vi "Main.vi"(10 "DAQ Type":enum16{"Hardware", "Simulation"}(ring), 11 "Module Admin":refnum<class "Delacor_lib_QMH_Module Admin.lvclass">) -> ()   [LabVIEW 2016, in "Oscilloscope.lvlib"]
doc: "This template is based off of the Queued Message Handler design pattern and the Queued Message Handler project template that ships with LabVIEW.\n\nThe main difference is that the queue is private to this module and communication between modules is performed via Broadcast and Request events.\n\nRequest events are wrapped in public API methods and are handled in the Event Handling Loop (EHL) of this VI. Any module can register for Broadcast events sent by this module. The EHL generates messages based on user interface actions.\n\nThe Message Handling Loop (MHL) processes messages generated by the EHL, or by other messages. The messages are string values, so new messages can be added easily to the Message Cases case structure in the MHL. Each message cluster can also provide an optional value for Message Data, which is a variant that can be converted to whatever message-specific data is required.\n_____\nBased on DQMH Project Template 6.1.0.94."
uses:
  Oscilloscope.lvlib
  <vilib>/Delacor/Delacor QMH/Libraries/Module Admin_class/Delacor_lib_QMH_Module Admin.lvclass
  Class/Agilent 3054A/Agilent 3054A.lvclass
  D:/common_ATE/Libraries/Oscilloscope/Class/Abstract/Abstract.lvclass
  Message Data.ctl
  Class/Abstract/Abstract.lvclass
  Module Data--cluster.ctl
  Scope Config Setting.ctl
  <vilib>/Delacor/Delacor QMH/Libraries/Message Queue_class/Delacor_lib_QMH_Message Queue.lvclass/Delacor_lib_QMH_Message Queue.ctl
  Stop Argument--cluster.ctl
  <vilib>/Delacor/Delacor QMH/Libraries/Module Admin_class/Delacor_lib_QMH_Module Admin.lvclass/Delacor_lib_QMH_Module Admin.ctl
  REQ Initialize Hardware Argument--cluster.ctl
  REQ Initialize Hardware (Reply Payload)--cluster.ctl
  REQ Auto setup Argument--cluster.ctl
  Close Ref Argument--cluster.ctl
  Acquire Waveform Argument--cluster.ctl
  Acquire Waveform (Reply Payload)--cluster.ctl
  REQ Channel Setting Argument--cluster.ctl
  REQ Configure DVM Argument--cluster.ctl
  REQ Read DVM Argument--cluster.ctl
  REQ Read DVM (Reply Payload)--cluster.ctl
  REQ Acq Waveform Argument--cluster.ctl
  REQ Retry Oscilloscope Argument--cluster.ctl
  <vilib>/Utility/miscctls.llb/LVPointTypeDef.ctl
  User Interface/Instrument Address Command.ctl
  <vilib>/Delacor/Delacor QMH/Libraries/Message Queue_class/Delacor_lib_QMH_Enqueue Message (Single).vi
  <vilib>/Delacor/Delacor QMH/Libraries/Module Admin_class/Delacor_lib_QMH_Get External Launch.vi
  <vilib>/Utility/error.llb/Error Cluster From Error Code.vi
  <vilib>/ErrorRing/Error Ring.xnode
  <vilib>/Delacor/Delacor QMH/Libraries/Message Queue_class/Delacor_lib_QMH_Message Queue.lvclass
  User Interface/User Interface.lvlib
  Error Log/Error Log.lvlib
panel:
  out "Channel":i32
  out "Waveform Data":waveform(dbl)(graph)
  out "error out":errorcluster
  out "Status":string
  in  "Simulate MHL Error":bool
  in  "Simulate EHL Error":bool
  # "Other QMH Modules communicate with this Module via its Public API (wrappers for its Request Events).\n\nThis Module communicates with other Modules via its Broadcast Events.\nAny module that wants to get these messages, just registers for this module's Broadcast events."
  # "This template is for the Delacor Modified Queued Message Handler design pattern.\n\nSee the block diagram for more information on how to use this template."
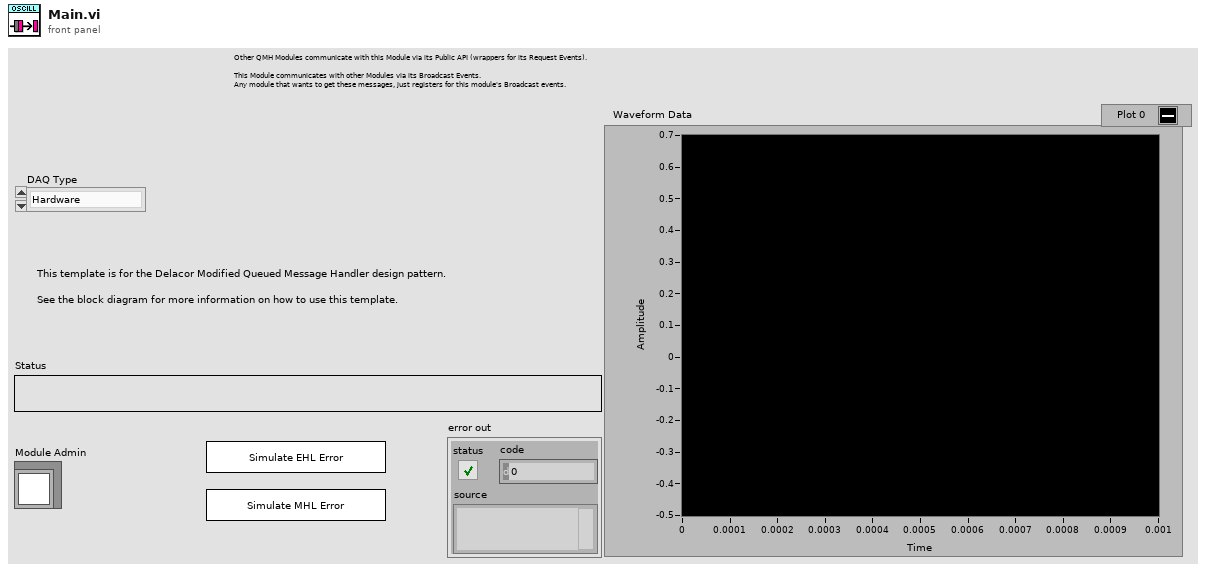
[diagram p1: front panel]
types:
  T1 = typedef "Oscilloscope.lvlib/Message Data.ctl" = cluster{"Message":string, "Data":waveform(dbl)}
  T2 = typedef "Oscilloscope.lvlib/Request Events--cluster.ctl" = cluster{"Stop Module":refnum<user-event>, "Show Panel":refnum<user-event>, "Hide Panel":refnum<user-event>, "Get Module Execution Status":refnum<user-event>, "Show Diagram":refnum<user-event>, "REQ Initialize Hardware":refnum<user-event>, "REQ Auto setup":refnum<user-event>, "Close Ref":refnum<user-event>, "Acquire Waveform":refnum<user-event>, "REQ Channel Setting":refnum<user-event>, "REQ Configure DVM":refnum<user-event>, "REQ Read DVM":refnum<user-event>, "REQ Acq Data":refnum<user-event>, "REQ Wakeup_helper_loop":refnum<user-event>, "REQ Acq Waveform":refnum<user-event>, "REQ Retry Oscilloscope":refnum<user-event>}
  T3 = enum32{"invalid lock state", "Not Locked", "Locked (No Password)", "Password-protected"}
  T4 = typedef "Oscilloscope.lvlib/Stop Argument--cluster.ctl" = cluster{"Origin":string, "Exit via Stop Module Req?":bool, "Wait for Module to stop?":bool}
  T5 = typedef "Oscilloscope.lvlib/REQ Initialize Hardware Argument--cluster.ctl" = cluster{"Connection Ref":variant, "Wait Notifier":refnum<notifier>, "wait for reply":bool}
  T6 = typedef "Oscilloscope.lvlib/REQ Auto setup Argument--cluster.ctl" = cluster{"Boolean":bool}
  T7 = typedef "Oscilloscope.lvlib/Close Ref Argument--cluster.ctl" = cluster{"Boolean":bool}
  T8 = typedef "Oscilloscope.lvlib/Acquire Waveform Argument--cluster.ctl" = cluster{"Channel":i32, "Wait Notifier":refnum<notifier>, "wait for reply":bool}
  T9 = typedef "Oscilloscope.lvlib/REQ Channel Setting Argument--cluster.ctl" = cluster{"Channel Setting":cluster{"Channel Name (0: Channel 1)":i32, "Coupling (1: DC)":i32, "Vertical Offset (0.0)":dbl, "Vertical Range (40.0 V)":dbl, "Probe Attenuation (1.0)":dbl, "Enable Channel (T: Enable)":bool, "Impedance (0: 1 MOhm)":i32, "Vertical Scale (5.0 V)":dbl, "Vertical Setting (1: Vertical Range)":i32}}
  T10 = typedef "Oscilloscope.lvlib/REQ Configure DVM Argument--cluster.ctl" = cluster{"DVM Setting":cluster{"DVM Channel":i32, "Enable DVM Analysis":bool, "Auto Range ":bool, "DVM Type":i32}}
  T11 = typedef "Oscilloscope.lvlib/REQ Read DVM Argument--cluster.ctl" = cluster{"Wait Notifier":refnum<notifier>, "wait for reply":bool}
  T12 = typedef "Oscilloscope.lvlib/REQ Acq Waveform Argument--cluster.ctl" = cluster{"Boolean":bool, "Channel":i32}
  T13 = typedef "Oscilloscope.lvlib/REQ Retry Oscilloscope Argument--cluster.ctl" = cluster{"Boolean":bool}
  T14 = typedef "User Interface.lvlib/Instrument Address Command.ctl" = enum16{"Init", "Read", "Write", "Close"}
  T15 = typedef "LVPointTypeDef.ctl" = cluster{"Horizontal":i16, "Vertical":i16}
  T16 = enum32{"Invalid", "Standard", "Closed", "Hidden", "Minimized", "Maximized"}
  T17 = typedef "Oscilloscope.lvlib/REQ Initialize Hardware (Reply Payload)--cluster.ctl" = cluster{"Connect?":bool, "error":errorcluster}
  T18 = typedef "Oscilloscope.lvlib/REQ Read DVM (Reply Payload)--cluster.ctl" = cluster{"3-digit DVM":dbl, "5-digit Frequency":dbl, "error":errorcluster}
  T19 = typedef "Oscilloscope.lvlib/Module Data--cluster.ctl" = cluster{"Status":string, "Abstract.lvclass":refnum<class "Abstract.lvclass">, "Inst_Path":path, "Scope":T20}
  T20 = typedef "Oscilloscope.lvlib/Scope Config Setting.ctl" = cluster{"Connection":cluster{"Ref":variant}, "Channel Setting":cluster{"Channel Name (0: Channel 1)":i32, "Coupling (1: DC)":i32, "Vertical Offset (0.0)":dbl, "Vertical Range (40.0 V)":dbl, "Probe Attenuation (1.0)":dbl, "Enable Channel (T: Enable)":bool, "Impedance (0: 1 MOhm)":i32, "Vertical Scale (5.0 V)":dbl, "Vertical Setting (1: Vertical Range)":i32}}
  T21 = cluster{"Channel Name (0: Channel 1)":i32, "Coupling (1: DC)":i32, "Vertical Offset (0.0)":dbl, "Vertical Range (40.0 V)":dbl, "Probe Attenuation (1.0)":dbl, "Enable Channel (T: Enable)":bool, "Impedance (0: 1 MOhm)":i32, "Vertical Scale (5.0 V)":dbl, "Vertical Setting (1: Vertical Range)":i32}
  T22 = cluster{"DVM Channel":i32, "Enable DVM Analysis":bool, "Auto Range ":bool, "DVM Type":i32}
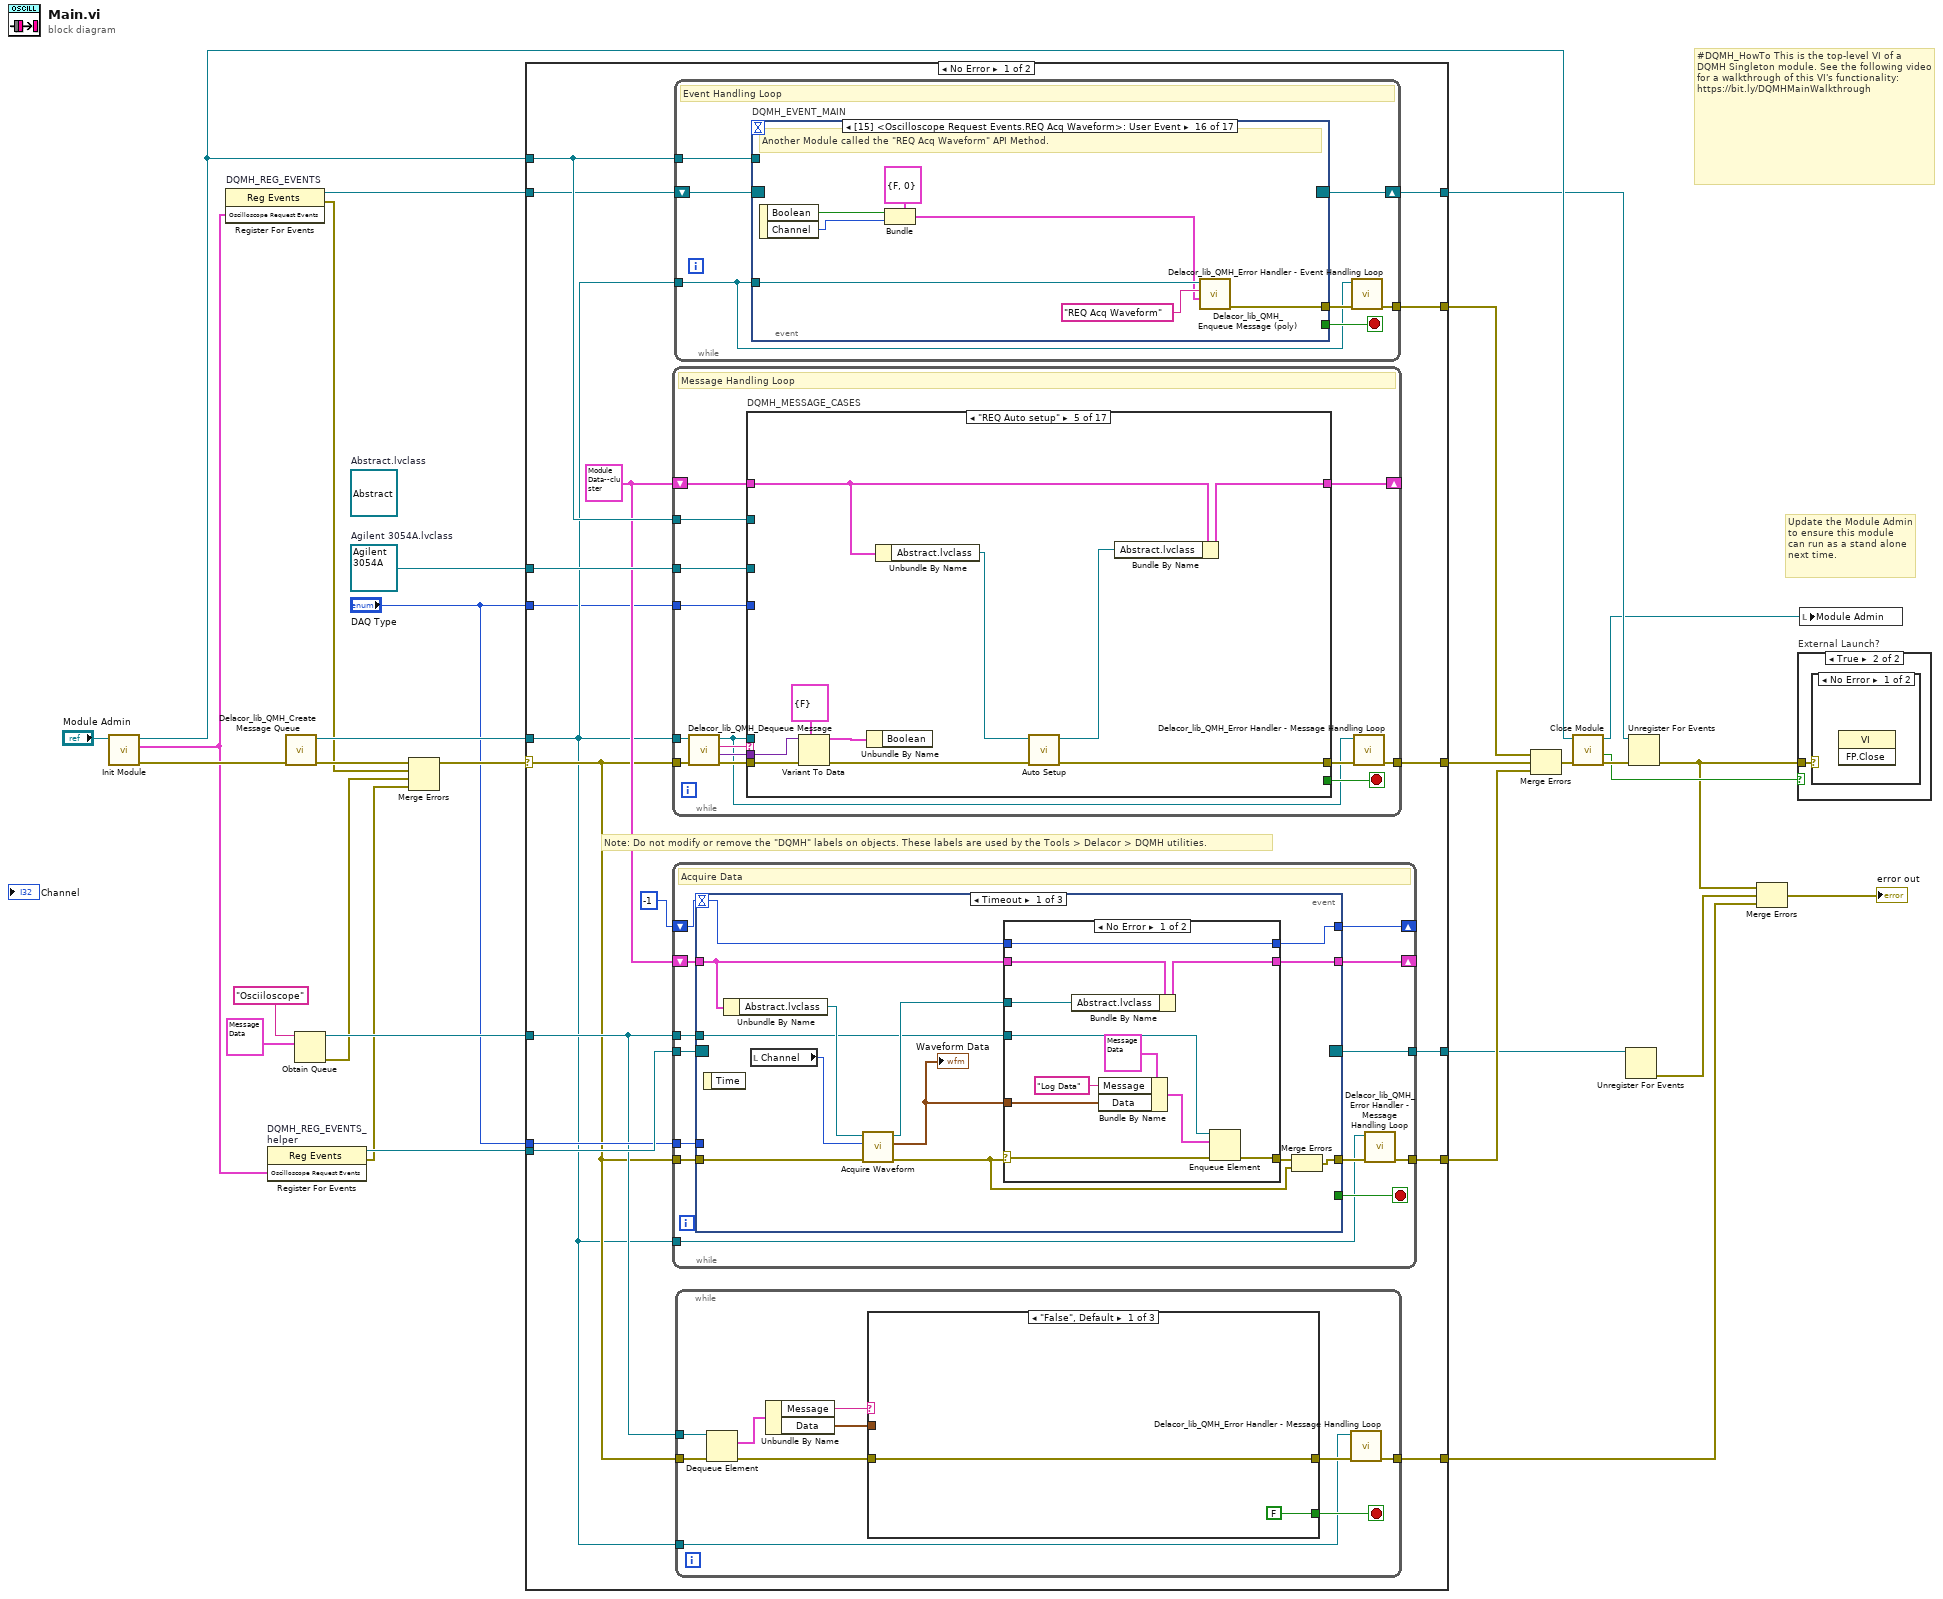
[diagram p0: block diagram]
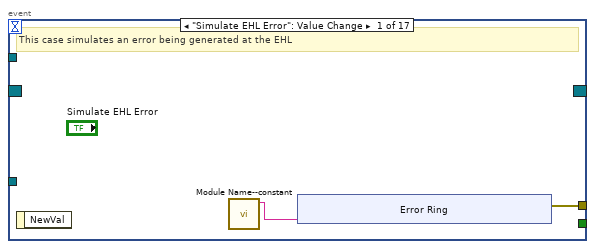
[diagram p2: hidden frame]
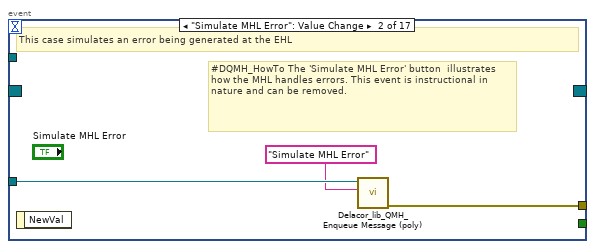
[diagram p3: hidden frame]
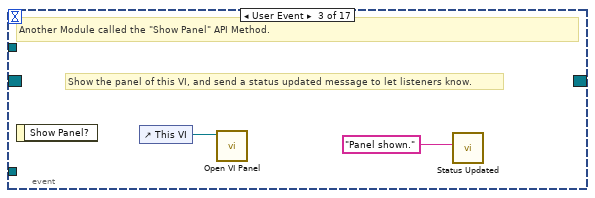
[diagram p4: hidden frame]
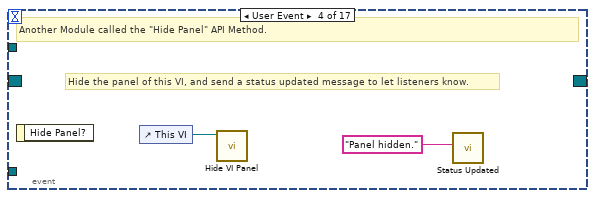
[diagram p5: hidden frame]
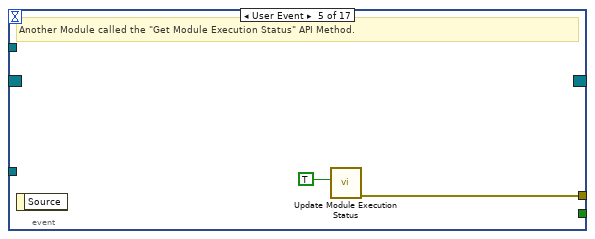
[diagram p6: hidden frame]
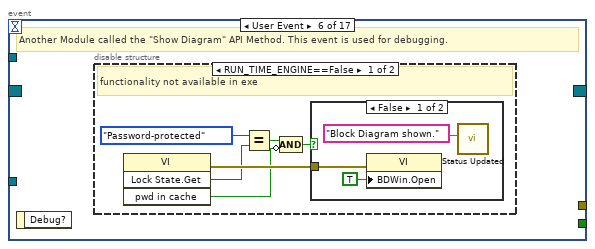
[diagram p7: hidden frame]
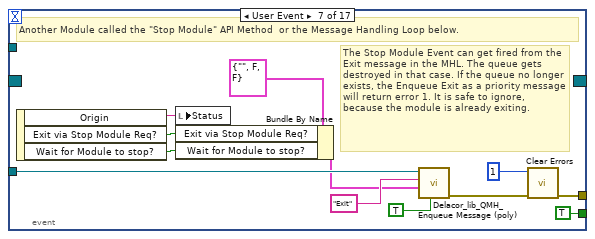
[diagram p10: hidden frame]
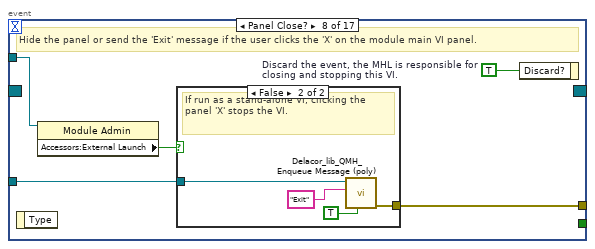
[diagram p11: hidden frame]
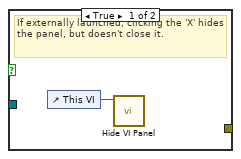
[diagram p12: hidden frame]
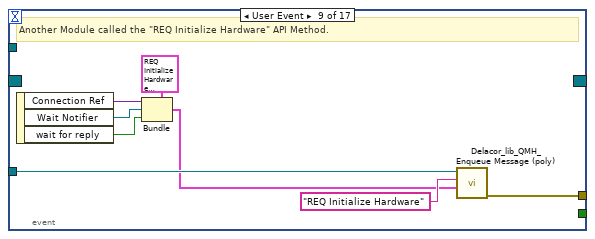
[diagram p13: hidden frame]
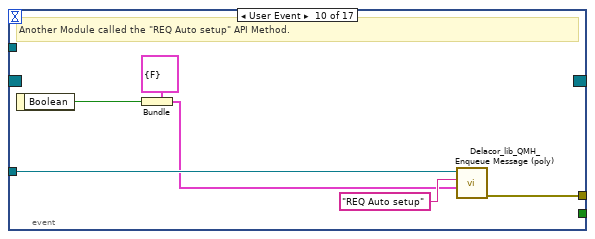
[diagram p14: hidden frame]
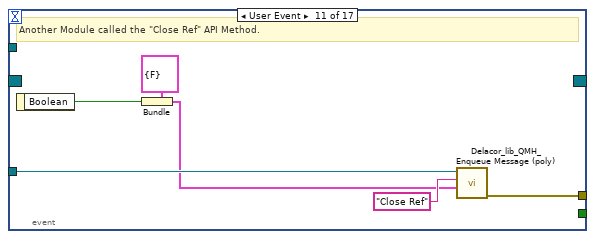
[diagram p15: hidden frame]
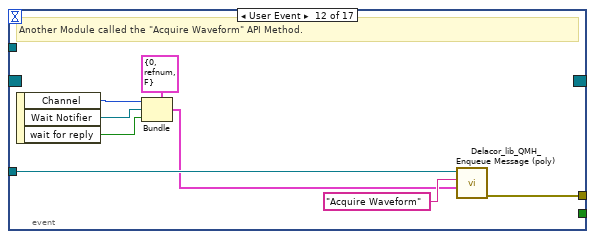
[diagram p16: hidden frame]
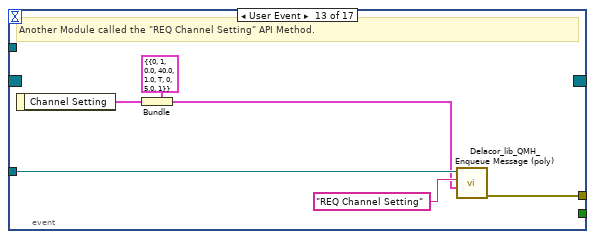
[diagram p17: hidden frame]
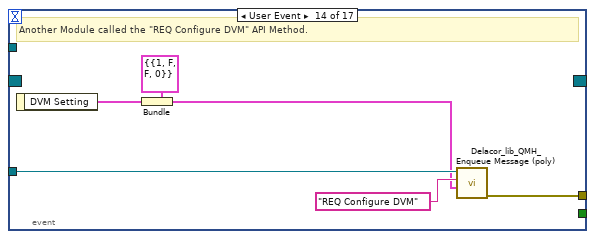
[diagram p18: hidden frame]
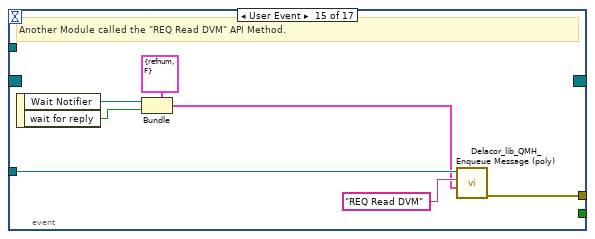
[diagram p19: hidden frame]
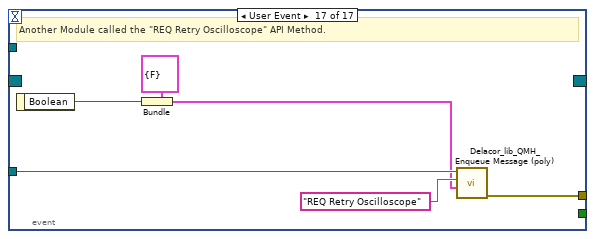
[diagram p20: hidden frame]
diagram:
  w16 = refnum<class "Agilent 3054A.lvclass"> refnum  # Agilent 3054A.lvclass
  (unwired) refnum<class "Abstract.lvclass"> refnum  # Abstract.lvclass
  # "#DQMH_HowTo This is the top-level VI of a DQMH Singleton module. See the following video for a walkthrough of this VI's functionality: https://bit.ly/DQMHMainWalkthrough"
  # "Update the Module Admin to ensure this module can run as a stand alone next time."
  n1 = call "Init Module.vi"("Singleton Module Admin in"="Module Admin") -> ("error out"=w29:errorcluster, "Oscilloscope Request Events"=w15:T2, "Singleton Module Admin out"=w23:refnum<class "Delacor_lib_QMH_Module Admin.lvclass">)  [unwired: 8 in]
  n2 = register-events "DQMH_REG_EVENTS"(w15) -> (reference out=w21:refnum<event-registration>, error out=w8:errorcluster)  [unwired: 2 in]
  n3 = register-events "DQMH_REG_EVENTS_helper"(w15) -> (reference out=w14:refnum<event-registration>, error out=w2:errorcluster)  [unwired: 2 in]
  n4 = call <vilib>:"Delacor_lib_QMH_Create Message Queue.vi"("error in"=w29) -> ("error out"=w25:errorcluster, "Message Queue"=w20:refnum<class "Delacor_lib_QMH_Message Queue.lvclass">)  [unwired: 9 in]
  n5 = Obtain Queue(name (unnamed)="Osciiloscope", element data type=T1 {"Message"="", "Data"={"t0"=timestamp(0 s since 1904-01-01), "dt"=1.0, "Y"=[]}}) -> (queue out=w5:refnum<queue>, error out=w3:errorcluster)  [unwired: 3 in, 1 out]
  n6 = Merge Errors(w25, w8, w3, w2) -> (w24:errorcluster)
  n7 = case shown="No Error" w24 {
    selector: w24 -> [w33 w461]
    tunnel: [w47 w460] -> w30
    tunnel: [w46 _] -> w27
    tunnel: w23 -> [w45 w464]
    tunnel: [w44 w463] -> w22
    tunnel: w21 -> [w43 w463]
    tunnel: w20 -> [w32 w462]
    tunnel: w16 -> [w42 _]
    tunnel: w14 -> [w40 _]
    tunnel: [w39 _] -> w13
    tunnel: [w38 _] -> w11
    tunnel: "DAQ Type" -> [w36 _]
    tunnel: w5 -> [w35 _]
    tunnel: [w34 _] -> w4
    tunnel: "DAQ Type" -> [w31 _]
    frame No Error {
      w37 = T19 {"Status"="", "Abstract.lvclass"=refnum, "Inst_Path"=path "", "Scope"={"Connection"={"Ref"=variant}, "Channel Setting"={"Channel Name (0: Channel 1)"=0, "Coupling (1: DC)"=1, "Vertical Offset (0.0)"=0.0, "Vertical Range (40.0 V)"=40.0, "Probe Attenuation (1.0)"=1.0, "Enable Channel (T: Enable)"=TRUE, "Impedance (0: 1 MOhm)"=0, "Vertical Scale (5.0 V)"=5.0, "Vertical Setting (1: Vertical Range)"=1}}} ("Data Cluster")
      # "Note: Do not modify or remove the \"DQMH\" labels on objects. These labels are used by the Tools > Delacor > DQMH utilities."
      n8 = while {
        tunnel: w32 -> [w168]
        shift-right: [w172] -> _
        shift-left: w37 -> [w173]
        tunnel: w33 -> [w176]
        tunnel: [w174] -> w47
        tunnel: w45 -> [w166]
        tunnel: w42 -> [w165]
        tunnel: w31 -> [w164]
        stop <- w171 stop-if-true
        # "Message Handling Loop"
        n9 = call-dynamic "Delacor_lib_QMH_Dequeue Message.vi"("error in"=w176, "Message Queue in"=w168) -> ("error out"=w175:errorcluster, "Message Data"=w169:variant, "Message"=w170:string, "Message Queue out"=w167:refnum<class "Delacor_lib_QMH_Message Queue.lvclass">)  [unwired: 6 in]
        n10 = case "DQMH_MESSAGE_CASES" shown="\"REQ Auto setup\"" w170 {
          selector: w170 -> [_ _ _ _ _ _ _ _ _ _ _ _ _ _ _ _ w379]
          tunnel: w167 -> [w184 _ _ _ _ _ _ _ _ _ _ _ _ _ w350 w371 _]
          tunnel: w175 -> [w180 w215 w217 w235 w247 w257 w268 w284 w296 w307 w322 w332 w334 w339 w357 w377 w381]
          tunnel: [w185 w208 w217 w222 w242 w253 w263 w275 w291 w301 w311 w331 w334 w338 w353 w374 w382] -> w177
          tunnel: w173 -> [w194 w214 w216 w227 w241 w252 w261 w274 w290 w300 w318 w330 w333 w336 w352 w370 w380]
          tunnel: [w193 w206 w216 w224 w239 w250 w259 w272 w288 w300 w309 w330 w333 w336 w352 w370 w380] -> w172
          tunnel: [_ _ _ _ _ _ _ _ _ _ _ _ _ _ _ w369 _] -> w171
          tunnel: w169 -> [_ _ _ w234 w245 w256 w267 w283 w295 w306 w321 _ _ _ w351 w368 _]
          tunnel: w166 -> [w195 _ _ _ _ _ _ _ _ _ _ _ _ _ w349 w363 _]
          tunnel: w165 -> [w187 _ _ _ _ _ _ _ _ _ _ _ _ _ _ _ _]
          tunnel: w164 -> [_ _ _ w223 _ _ _ _ _ _ w315 _ _ _ _ _ _]
          frame "Initialize" {
            w189 = "Initial Message" ("Initial Message")
            # "Initialize - Any operation that needs to be done before the module can receive messages. Synchronize Caller Events.vi will inform Start Module.vi that the module has launched and is ready to receive messages. Module Did Init.vi will broadcast that the module initialized."
            n11 = call "Synchronize Caller Events.vi"("error in (no error)"=w180, "Singleton Module Admin in"=w195) -> ("error out"=w183:errorcluster, "Singleton Module Admin out"=w190:refnum<class "Delacor_lib_QMH_Module Admin.lvclass">)  [unwired: 8 in]
            n12 = property class="Module Admin"(reference=w190) -> ("Accessors:External Launch"=w199:bool)  [unwired: 1 in, 2 out]
            n13 = property on="Pane" class="Pane"("Origin"=T15 {"Horizontal"=0, "Vertical"=0}) -> ()  [unwired: 2 in, 2 out]
            n14 = call "Module Name--constant.vi"() -> ("Module Name"=w191:string)  [unwired: 11 in]
            n15 = call "Module Did Init.vi"("error in (no error)"=w183, "Initialized?"=TRUE, "Origin"=w191) -> ()  [unwired: 8 in, 1 out]
            n16 = call "Instrument Address.vi"("Command"=Instrument_Address_Command."Init", "error in (no error)"=w180, "name or relative path"="Instrument.ini") -> ("error out"=w179:errorcluster, "path_out"=w178:path)  [unwired: 6 in, 1 out]
            n17 = Select(t=T16."Hidden" ("State"), s=w199, f=T16."Standard" ("State")) -> (s? t:f=w196:T16)
            n18 = call "Module Name--constant.vi"() -> ("Module Name"=w202:string)  [unwired: 11 in]
            n19 = property class="VI"("Front Panel.Title"=w202) -> (reference out=w201:refnum<vi>, error out=w204:errorcluster)  [unwired: 2 in]
            n20 = Bundle By Name(cluster=w194, "Status"=w189, "Abstract.lvclass"=w187, "Inst_Path"=w178) -> (w193:T19)
            n21 = invoke class="VI" method="FP.Open"(reference=w201, error in=w204, "State"=w196) -> (reference out=w200:refnum<vi>, error out=w203:errorcluster)  [unwired: 2 in, 3 out]
            n22 = call-poly <vilib>:"Delacor_lib_QMH_Enqueue Message (poly).vi"("error in"=w179, "Message"="REQ Inst Address", "Message Queue in"=w184) -> ("error out"=w185:errorcluster)  [unwired: 7 in, 1 out]
            n23 = invoke class="VI" method="FP.Center"(reference=w200, error in=w203) -> ()  [unwired: 1 in, 3 out]
            "Status" <- w189
          }
          frame "REQ Inst Address" {
            n24 = Unbundle By Name(w214) -> ("Inst_Path"=w212:path)
            n25 = call "Instrument Address.vi"("Command"=Instrument_Address_Command."Read", "error in (no error)"=w215, "path_in"=w212) -> ("error out"=w209:errorcluster, "Instrument Parameter"=w211:string[][])  [unwired: 6 in, 1 out]
            n26 = Index Array(array=w211, index (row)=3) -> (element=w207:string[])  [unwired: 1 in]
            n27 = call "Update Inst Config.vi"("error in (no error)"=w209, "Data In"=w207) -> ("error out"=w208:errorcluster, "Scope"=w205:T20)  [unwired: 8 in]
            n28 = Bundle By Name(cluster=w214, "Scope"=w205) -> (w206:T19)
          }
          frame "---Module Specific---" {
            # "Separator -- The following cases handle messages specific to this Module."
          }
          frame "REQ Initialize Hardware" {
            n29 = Variant To Data(error in=w235, type=T5 {"Connection Ref"=variant, "Wait Notifier"=refnum, "wait for reply"=FALSE} ("REQ Initialize Hardware Argument"), Variant=w234) -> (data=w232:T5, error out=w225:errorcluster)
            n30 = Unbundle By Name(w227) -> ("Abstract.lvclass"=w226:refnum<class "Abstract.lvclass">, "Scope.Connection.Ref"=w218:variant)
            n31 = Unbundle By Name(w232) -> ("Wait Notifier"=w231:refnum<notifier>, "wait for reply"=w230:bool)
            n32 = call-dynamic "Initialize Hardware.vi"("error in (no error)"=w225, "DAQ Type"=w223, "Connection Ref"=w218, "Abstract in"=w226) -> ("error out"=w222:errorcluster, "Abstract out"=w219:refnum<class "Abstract.lvclass">)  [unwired: 6 in]
            n33 = Unbundle By Name(w222) -> ("status"=w221:bool)
            n34 = Bundle By Name(cluster=w227, "Abstract.lvclass"=w219) -> (w224:T19)
            n35 = Not(x=w221) -> (.not. x?=w220:bool)
            n36 = Bundle By Name(cluster=T17 {"Connect?"=FALSE, "error"={"status"=FALSE, "code"=0, "source"=""}} ("REQ Initialize Hardware (Reply Payload)"), "Connect?"=w220) -> (w229:T17)
            n37 = case shown="True" w230 {
              tunnel: w231 -> [_ w237]
              tunnel: w229 -> [_ w236]
              frame False {
              }
              frame True {
                n38 = Send Notification(notification=w236, notifier=w237) -> ()  [unwired: 1 in, 2 out]
              }
            }
          }
          frame "REQ Auto setup" {
            n39 = Variant To Data(error in=w247, type=T6 {"Boolean"=FALSE} ("REQ Auto setup Argument"), Variant=w245) -> (data=w243:T6, error out=w246:errorcluster)
            n40 = Unbundle By Name(w243) -> ()  [unwired: 1 out]
            n41 = Unbundle By Name(w241) -> ("Abstract.lvclass"=w240:refnum<class "Abstract.lvclass">)
            n42 = call-dynamic "Auto Setup.vi"("error in (no error)"=w246, "Abstract in"=w240) -> ("error out"=w242:errorcluster, "Abstract out"=w238:refnum<class "Abstract.lvclass">)  [unwired: 8 in]
            n43 = Bundle By Name(cluster=w241, "Abstract.lvclass"=w238) -> (w239:T19)
          }
          frame "REQ Channel Setting" {
            n44 = Variant To Data(error in=w257, type=T9 {"Channel Setting"={"Channel Name (0: Channel 1)"=0, "Coupling (1: DC)"=1, "Vertical Offset (0.0)"=0.0, "Vertical Range (40.0 V)"=40.0, "Probe Attenuation (1.0)"=1.0, "Enable Channel (T: Enable)"=TRUE, "Impedance (0: 1 MOhm)"=0, "Vertical Scale (5.0 V)"=5.0, "Vertical Setting (1: Vertical Range)"=1}} ("REQ Channel Setting Argument"), Variant=w256) -> (error out=w254:errorcluster)  [unwired: 1 out]
            n45 = Unbundle By Name(w252) -> ("Abstract.lvclass"=w251:refnum<class "Abstract.lvclass">, "Scope.Channel Setting"=w248:T21)
            n46 = call-dynamic "Configure Channel.vi"("error in (no error)"=w254, "Channel Setting"=w248, "Abstract in"=w251) -> ("error out"=w253:errorcluster, "Abstract out"=w249:refnum<class "Abstract.lvclass">)  [unwired: 7 in]
            n47 = Bundle By Name(cluster=w252, "Abstract.lvclass"=w249) -> (w250:T19)
          }
          frame "REQ Configure DVM" {
            n48 = Variant To Data(error in=w268, type=T10 {"DVM Setting"={"DVM Channel"=1, "Enable DVM Analysis"=FALSE, "Auto Range "=FALSE, "DVM Type"=0}} ("REQ Configure DVM Argument"), Variant=w267) -> (data=w265:T10, error out=w264:errorcluster)
            n49 = Unbundle By Name(w265) -> ("DVM Setting"=w262:T22)
            n50 = Unbundle By Name(w261) -> ("Abstract.lvclass"=w260:refnum<class "Abstract.lvclass">)
            n51 = call-dynamic "Configure DVM Setting.vi"("error in (no error)"=w264, "DVM Setting"=w262, "Abstract in"=w260) -> ("error out"=w263:errorcluster, "Abstract out"=w258:refnum<class "Abstract.lvclass">)  [unwired: 7 in]
            n52 = Bundle By Name(cluster=w261, "Abstract.lvclass"=w258) -> (w259:T19)
          }
          frame "REQ Read DVM" {
            n53 = Variant To Data(error in=w284, type=T11 {"Wait Notifier"=refnum, "wait for reply"=FALSE} ("REQ Read DVM Argument"), Variant=w283) -> (data=w281:T11, error out=w276:errorcluster)
            n54 = Unbundle By Name(w281) -> ("Wait Notifier"=w280:refnum<notifier>, "wait for reply"=w279:bool)
            n55 = Unbundle By Name(w274) -> ("Abstract.lvclass"=w273:refnum<class "Abstract.lvclass">)
            n56 = call-dynamic "Read DVM.vi"("error in (no error)"=w276, "Abstract in"=w273) -> ("error out"=w275:errorcluster, "5-digit Frequency"=w269:dbl, "3-digit DVM"=w270:dbl, "Abstract out"=w271:refnum<class "Abstract.lvclass">)  [unwired: 6 in]
            n57 = Bundle By Name(cluster=T18 {"3-digit DVM"=0.0, "5-digit Frequency"=0.0, "error"={"status"=FALSE, "code"=0, "source"=""}} ("REQ Read DVM (Reply Payload)"), "3-digit DVM"=w270, "5-digit Frequency"=w269) -> (w278:T18)
            n58 = Bundle By Name(cluster=w274, "Abstract.lvclass"=w271) -> (w272:T19)
            n59 = case shown="True" w279 {
              tunnel: w280 -> [_ w286]
              tunnel: w278 -> [_ w285]
              frame False {
              }
              frame True {
                n60 = Send Notification(notification=w285, notifier=w286) -> ()  [unwired: 1 in, 2 out]
              }
            }
          }
          frame "Close Ref" {
            n61 = Variant To Data(error in=w296, type=T7 {"Boolean"=FALSE} ("Close Ref Argument"), Variant=w295) -> (data=w293:T7, error out=w292:errorcluster)
            n62 = Unbundle By Name(w290) -> ("Abstract.lvclass"=w289:refnum<class "Abstract.lvclass">)
            n63 = Unbundle By Name(w293) -> ()  [unwired: 1 out]
            n64 = call-dynamic "Close Ref.vi"("error in (no error)"=w292, "Abstract in"=w289) -> ("error out"=w291:errorcluster, "Abstract out"=w287:refnum<class "Abstract.lvclass">)  [unwired: 8 in]
            n65 = Bundle By Name(cluster=w290, "Abstract.lvclass"=w287) -> (w288:T19)
          }
          frame "REQ Acq Waveform" {
            n66 = Variant To Data(error in=w307, type=T12 {"Boolean"=FALSE, "Channel"=0} ("REQ Acq Waveform Argument"), Variant=w306) -> (data=w304:T12, error out=w303:errorcluster)
            n67 = Unbundle By Name(w300) -> ("Abstract.lvclass"=w299:refnum<class "Abstract.lvclass">)
            n68 = Unbundle By Name(w304) -> ("Channel"=w302:i32)
            n69 = To Variant(anything=w299) -> (Variant=w297:variant)
            n70 = call "REQ Wakeup_helper_loop.vi"("error in"=w303, "Channel"=w302, "Timeout"=0, "Data"=w297) -> ("error out"=w301:errorcluster)  [unwired: 7 in]
          }
          frame "REQ Retry Oscilloscope" {
            n71 = Unbundle By Name(w318) -> ("Abstract.lvclass"=w317:refnum<class "Abstract.lvclass">, "Scope.Connection.Ref"=w316:variant)
            n72 = Variant To Data(error in=w322, type=T13 {"Boolean"=FALSE} ("REQ Retry Oscilloscope Argument"), Variant=w321) -> (error out=w319:errorcluster)  [unwired: 1 out]
            n73 = call-dynamic "Initialize Hardware.vi"("error in (no error)"=w319, "DAQ Type"=w315, "Connection Ref"=w316, "Abstract in"=w317) -> ("error out"=w310:errorcluster, "Abstract out"=w308:refnum<class "Abstract.lvclass">)  [unwired: 6 in]
            n74 = local read "Channel"() -> (w313:i32)
            n75 = Bundle By Name(cluster=w318, "Abstract.lvclass"=w308) -> (w309:T19)
            n76 = case shown="No Error" w310 {
              selector: w310 -> [w327 _]
              tunnel: [w328 w329] -> w314
              tunnel: w308 -> [w326 _]
              tunnel: w313 -> [w325 _]
              frame No Error {
                n77 = To Variant(anything=w326) -> (Variant=w323:variant)
                n78 = call "REQ Wakeup_helper_loop.vi"("error in"=w327, "Channel"=w325, "Timeout"=0, "Data"=w323) -> ("error out"=w328:errorcluster)  [unwired: 7 in]
              }
              frame Error {
                n79 = call "REQ Retry Oscilloscope.vi"() -> ("error out"=w329:errorcluster)  [unwired: 11 in]
              }
            }
            n80 = Wait (ms)(milliseconds to wait=u32 2000) -> ()  [unwired: 1 out]
            n81 = Merge Errors(w310, w314) -> (w311:errorcluster)
          }
          frame "---Copy This Frame---" {
            # "Duplicate this frame when creating new messages.  Change this comment in the duplicated frame to describe this message."
            n82 = Merge Errors(w332) -> (w331:errorcluster)
          }
          frame "---Exit and Error Handling---" {
            # "Separator - The following cases handle errors and exit messages."
          }
          frame "Simulate MHL Error" {
            # "#DQMH_HowTo The 'Simulate MHL Error' button  illustrates how the MHL handles errors. This event is instructional in nature and can be removed."
            # "Simulate an error occurring at the MHL"
            n83 = call "Module Name--constant.vi"() -> ("Module Name"=w335:string)  [unwired: 11 in]
            n84 = xnode "Error Ring"("parameter 0"=w335) -> ("error out"=w337:errorcluster)
            n85 = Merge Errors(w339, w337) -> (w338:errorcluster)
          }
          frame "Error" {
            # "Error - Check the error message data and respond accordingly. This message is sent by the \"Error Handler\" VIs at the end of each loop in this application."
            n86 = property class="Module Admin"(reference=w349) -> ("Accessors:External Launch"=w348:bool)  [unwired: 1 in, 2 out]
            n87 = Variant To Data(error in=w357, type=errorcluster {"status"=FALSE, "code"=0, "source"=""} ("error constant"), Variant=w351) -> (data=w347:errorcluster, error out=w355:errorcluster)
            n88 = call "Error Reported.vi"("Error"=w347) -> ()  [unwired: 10 in, 1 out]
            n89 = call "REQ Log Error.vi"("error in (no error)"=w347) -> ()  [unwired: 10 in, 1 out]
            n90 = case shown="False" w348 {
              tunnel: [w362 _] -> w354
              tunnel: w350 -> [w360 _]
              tunnel: w347 -> [w361 _]
              frame False {
                n91 = call <vilib>:"Simple Error Handler.vi"("error in (no error)"=w361) -> ()  [unwired: 4 in, 5 out]
                n92 = call-poly <vilib>:"Delacor_lib_QMH_Enqueue Message (poly).vi"("Priority Message? (F)"=TRUE, "Message"="REQ Reconnect", "Message Queue in"=w360) -> ("error out"=w362:errorcluster)  [unwired: 7 in, 1 out]
              }
              frame True {
                # "If the module was launched externally, calling the Error Reported broadcast VI is the only action performed by the \"Error\" message. The module's caller can then process the error appropriately."
              }
            }
            n93 = Merge Errors(w355, w354) -> (w353:errorcluster)
            n94 = local write "error out"(w353) -> ()
          }
          frame "Exit" {
            w367 = 91  # 91: not all Exit messages will have an argument
            w369 = TRUE  # Stop the VI
            # "Release the message queue reference"
            # "#CodeNeeded - Add any required cleanup code here"
            # "Exit - Exit the application."
            n95 = Variant To Data(error in=w377, type=T4 {"Origin"="", "Exit via Stop Module Req?"=FALSE, "Wait for Module to stop?"=FALSE} ("Stop Argument"), Variant=w368) -> (data=w365:T4, error out=w373:errorcluster)
            n96 = call <vilib>:"Clear Errors.vi"("error in (no error)"=w373, "specific error code to clear (0: all)"=w367) -> ("error out"=w376:errorcluster)  [unwired: 4 in, 1 out]
            n97 = control-ref of="This VI"() -> (w364:refnum<vi>)
            n98 = call-dynamic "Delacor_lib_QMH_Release Message Queue.vi"("error in"=w376, "Message Queue"=w371) -> ("error out"=w375:errorcluster)  [unwired: 9 in]
            n99 = call "Handle Exit.vi"("Stop Argument"=w365, "Admin in"=w363, "VI reference"=w364) -> ("error out"=w372:errorcluster)  [unwired: 7 in, 1 out]
            n100 = Merge Errors(w375, w372) -> (w374:errorcluster)
          }
          frame Default {
            # "'Default' case only runs if there is a message that isn't defined in any of the other cases.  Output a programming error."
            n101 = call "Module Name--constant.vi"() -> ("Module Name"=w378:string)  [unwired: 11 in]
            n102 = xnode "Error Ring"("parameter 0"=w379, "parameter 1"=w378) -> ("error out"=w383:errorcluster)
            n103 = Merge Errors(w381, w383) -> (w382:errorcluster)
          }
        }
        n104 = call-dynamic "Delacor_lib_QMH_Error Handler - Message Handling Loop.vi"("error in"=w177, "Message Queue in"=w167) -> ("dup error in"=w174:errorcluster)  [unwired: 8 in, 1 out]
      }
      n105 = while {
        shift-right: [w413] -> _
        shift-left: -1 -> [w420]
        tunnel: w33 -> [w418]
        tunnel: [w409] -> w39
        tunnel: w40 -> [w419]
        tunnel: [w416] -> w38
        shift-right: [w414] -> _
        shift-left: w37 -> [w415]
        tunnel: w36 -> [w412]
        tunnel: w35 -> [w411]
        tunnel: w32 -> [w408]
        stop <- w417 stop-if-true
        # "Acquire Data"
        n106 = event shown="[0] Timeout" {
          selector: w419 -> [_ _ _]
          dyn-events: [_ _ _] -> w416
          timeout: w420 -> [w431 _ w452]
          tunnel: w418 -> [w433 w451 w454]
          tunnel: [_ _ TRUE] -> w417
          tunnel: [w422 w451 w453] -> w410
          tunnel: w415 -> [w428 _ _]
          tunnel: [w429 _ _] -> w414
          tunnel: [w430 _ w452] -> w413
          tunnel: w412 -> [_ _ _]
          tunnel: w411 -> [w424 _ w455]
          event Timeout {
            n107 = event-data() -> ()  [unwired: 1 in, 1 out]
            n108 = Unbundle By Name(w428) -> ("Abstract.lvclass"=w432:refnum<class "Abstract.lvclass">)
            n109 = local read "Channel"() -> (w426:i32)
            n110 = call-dynamic "Acquire Waveform.vi"("error in (no error)"=w433, "Channel"=w426, "Abstract in"=w432) -> ("error out"=w421:errorcluster, "Waveform Data"=w423:waveform(dbl), "Abstract out"=w427:refnum<class "Abstract.lvclass">)  [unwired: 6 in]
            "Waveform Data" <- w423
            n111 = case shown="No Error" w421 {
              selector: w421 -> [w440 _]
              tunnel: w431 -> [w444 _]
              tunnel: [w444 -1] -> w430
              tunnel: [w442 w448] -> w429
              tunnel: w428 -> [w443 w449]
              tunnel: w427 -> [w441 w447]
              tunnel: [w439 w445] -> w425
              tunnel: w424 -> [w438 _]
              tunnel: w423 -> [w434 _]
              frame No Error {
                n112 = Bundle By Name(cluster=w443, "Abstract.lvclass"=w441) -> (w442:T19)
                n113 = Bundle By Name(cluster=T1 {"Message"="", "Data"={"t0"=timestamp(0 s since 1904-01-01), "dt"=1.0, "Y"=[]}}, "Message"="Log Data", "Data"=w434) -> (w436:T1)
                n114 = Enqueue Element(queue=w438, element=w436, error in (no error)=w440) -> (error out=w439:errorcluster)  [unwired: 1 in, 2 out]
              }
              frame Error {
                n115 = Bundle By Name(cluster=w449, "Abstract.lvclass"=w447) -> (w448:T19)
                n116 = call "Close Ref.vi"() -> ("error out"=w446:errorcluster)  [unwired: 11 in]
                n117 = call "REQ Retry Oscilloscope.vi"("error in"=w446) -> ("error out"=w445:errorcluster)  [unwired: 10 in]
              }
            }
            n118 = Merge Errors(w425, w421) -> (w422:errorcluster)
          }
          event User Event {
            n119 = event-data() -> ()  [unwired: 1 in, 1 out]
          }
          event User Event {
            n120 = event-data() -> ()  [unwired: 1 in, 1 out]
            n121 = Bundle By Name(cluster=T1 {"Message"="", "Data"={"t0"=timestamp(0 s since 1904-01-01), "dt"=1.0, "Y"=[]}}, "Message"="Stop") -> (w457:T1)
            n122 = Enqueue Element(queue=w455, element=w457, error in (no error)=w454) -> (error out=w453:errorcluster)  [unwired: 1 in, 2 out]
          }
        }
        n123 = call-dynamic "Delacor_lib_QMH_Error Handler - Message Handling Loop.vi"("error in"=w410, "Message Queue in"=w408) -> ("dup error in"=w409:errorcluster)  [unwired: 8 in, 1 out]
      }
      n124 = while {
        tunnel: w32 -> [w48]
        shift-right: [w51] -> w44
        shift-left: w43 -> [w52]
        tunnel: [w53] -> w46
        tunnel: w45 -> [w49]
        stop <- w50 stop-if-true
        # "Event Handling Loop"
        n125 = event "DQMH_EVENT_MAIN" shown="[15] <Oscilloscope Request Events.REQ Acq Waveform>: User Event" {
          selector: w52 -> [_ _ _ _ _ _ _ _ _ _ _ _ _ _ _ _ _]
          dyn-events: [_ _ _ _ _ _ _ _ _ _ _ _ _ _ _ _ _] -> w51
          timeout: _ -> [_ _ _ _ _ _ _ _ _ _ _ _ _ _ _ _ _]
          tunnel: [_ _ _ _ _ _ TRUE ("Discard?") _ _ _ _ _ _ _ _ _ _] -> w50
          tunnel: w48 -> [_ w65 _ _ _ _ w89 w96 w111 w117 w123 w131 w137 w143 w150 w157 w163]
          tunnel: [w56 w66 _ _ w72 _ w92 w98 w104 w112 w118 w126 w132 w138 w144 w152 w158] -> w54
          tunnel: w49 -> [_ _ _ _ _ _ _ w95 _ _ _ _ _ _ _ _ _]
          event "Simulate EHL Error": Value Change {
            # "This case simulates an error being generated at the EHL"
            n126 = event-data() -> ()  [unwired: 1 in, 1 out]
            n127 = call "Module Name--constant.vi"() -> ("Module Name"=w55:string)  [unwired: 11 in]
            n128 = xnode "Error Ring"("parameter 0"=w55) -> ("error out"=w56:errorcluster)
          }
          event "Simulate MHL Error": Value Change {
            # "#DQMH_HowTo The 'Simulate MHL Error' button  illustrates how the MHL handles errors. This event is instructional in nature and can be removed."
            # "This case simulates an error being generated at the EHL"
            n129 = event-data() -> ()  [unwired: 1 in, 1 out]
            n130 = call-poly <vilib>:"Delacor_lib_QMH_Enqueue Message (poly).vi"("Message"="Simulate MHL Error", "Message Queue in"=w65) -> ("error out"=w66:errorcluster)  [unwired: 8 in, 1 out]
          }
          event User Event {
            # "Show the panel of this VI, and send a status updated message to let listeners know."
            # "Another Module called the \"Show Panel\" API Method."
            n131 = event-data() -> ()  [unwired: 1 in, 1 out]
            n132 = control-ref of="This VI"() -> (w68:refnum<vi>)
            n133 = call "Open VI Panel.vi"("VI"=w68) -> ()  [unwired: 10 in, 1 out]
            n134 = call "Status Updated.vi"("Status"="Panel shown." ("format string")) -> ()  [unwired: 10 in, 1 out]
          }
          event User Event {
            # "Hide the panel of this VI, and send a status updated message to let listeners know."
            # "Another Module called the \"Hide Panel\" API Method."
            n135 = event-data() -> ()  [unwired: 1 in, 1 out]
            n136 = control-ref of="This VI"() -> (w70:refnum<vi>)
            n137 = call "Hide VI Panel.vi"("VI"=w70) -> ()  [unwired: 10 in, 1 out]
            n138 = call "Status Updated.vi"("Status"="Panel hidden." ("format string")) -> ()  [unwired: 10 in, 1 out]
          }
          event User Event {
            # "Another Module called the \"Get Module Execution Status\" API Method."
            n139 = event-data() -> ()  [unwired: 1 in, 1 out]
            n140 = call "Update Module Execution Status.vi"("Running?"=TRUE) -> ("error out"=w72:errorcluster)  [unwired: 10 in]
          }
          event User Event {
            # "Another Module called the \"Show Diagram\" API Method. This event is used for debugging."
            n141 = event-data() -> ()  [unwired: 1 in, 1 out]
            n142 = disable-structure shown="RUN_TIME_ENGINE==False" {
              frame condition #0 (active) {
                # "functionality not available in exe"
                n143 = invoke class="VI" method="Lock State.Get"() -> (error out=w78:errorcluster, "Get Lock State"=w77:T3, "pwd in cache"=w74:bool)  [unwired: 4 in, 1 out]
                n144 = Equal?(x=T3."Password-protected", y=w77) -> (x = y?=w75:bool)
                n145 = Compound Arithmetic op=AND(w75, invert w74) -> (w73:bool)
                n146 = case shown="False" w73 {
                  tunnel: w78 -> [w81 _]
                  frame False {
                    n147 = property class="VI"(error in=w81, "BDWin.Open"=TRUE ("Block Diagram Window:Open")) -> ()  [unwired: 1 in, 2 out]
                    n148 = call "Status Updated.vi"("Status"="Block Diagram shown." ("format string")) -> ()  [unwired: 10 in, 1 out]
                  }
                  frame True {
                    # "Password-protected VI, and the password is not in the cache. Do not show the diagram."
                  }
                }
              }
              frame condition #1 {
              }
            }
          }
          event User Event {
            # "The Stop Module Event can get fired from the Exit message in the MHL. The queue gets destroyed in that case. If the queue no longer exists, the Enqueue Exit as a priority message will return error 1. It is safe to ignore, because the module is already exiting."
            # "Another Module called the \"Stop Module\" API Method  or the Message Handling Loop below."
            n149 = event-data() -> ("Origin"=w88:string, "Exit via Stop Module Req?"=w84:bool, "Wait for Module to stop?"=w83:bool)  [unwired: 1 in]
            n150 = local write "Status"(w88) -> ()
            n151 = Bundle By Name(cluster=T4 {"Origin"="", "Exit via Stop Module Req?"=FALSE, "Wait for Module to stop?"=FALSE} ("Stop Argument"), "Exit via Stop Module Req?"=w84, "Wait for Module to stop?"=w83) -> (w82:T4)
            n152 = call-poly <vilib>:"Delacor_lib_QMH_Enqueue Message (poly).vi"("Priority Message? (F)"=TRUE, "Message Data"=w82, "Message"="Exit", "Message Queue in"=w89) -> ("error out"=w93:errorcluster)  [unwired: 6 in, 1 out]
            n153 = call <vilib>:"Clear Errors.vi"("error in (no error)"=w93, "specific error code to clear (0: all)"=1) -> ("error out"=w92:errorcluster)  [unwired: 4 in, 1 out]
          }
          event Panel Close? {
            w97 = TRUE  # Discard the event, the MHL is responsible for closing and stopping this VI.
            # "Hide the panel or send the 'Exit' message if the user clicks the 'X' on the module main VI panel."
            n154 = event-data() -> ()  [unwired: 1 in, 1 out]
            n155 = property class="Module Admin"(reference=w95) -> ("Accessors:External Launch"=w94:bool)  [unwired: 1 in, 2 out]
            n156 = case shown="False" w94 {
              tunnel: w96 -> [_ w102]
              tunnel: [_ w103] -> w98
              frame True {
                # "If externally launched, clicking the 'X' hides the panel, but doesn't close it."
                n157 = control-ref of="This VI"() -> (w99:refnum<vi>)
                n158 = call "Hide VI Panel.vi"("VI"=w99) -> ()  [unwired: 10 in, 1 out]
              }
              frame False {
                # "If run as a stand-alone VI, clicking the panel 'X' stops the VI."
                n159 = call-poly <vilib>:"Delacor_lib_QMH_Enqueue Message (poly).vi"("Priority Message? (F)"=TRUE, "Message"="Exit", "Message Queue in"=w102) -> ("error out"=w103:errorcluster)  [unwired: 7 in, 1 out]
              }
            }
            n160 = event-data("Discard?"=w97) -> ()  [unwired: 1 in, 1 out]
          }
          event User Event {
            # "Another Module called the \"REQ Initialize Hardware\" API Method."
            n161 = event-data() -> ("Connection Ref"=w107:variant, "Wait Notifier"=w106:refnum<notifier>, "wait for reply"=w105:bool)  [unwired: 1 in]
            n162 = Bundle(cluster=T5 {"Connection Ref"=variant, "Wait Notifier"=refnum, "wait for reply"=FALSE} ("REQ Initialize Hardware Argument"), "Connection Ref"=w107, "Wait Notifier"=w106, "wait for reply"=w105) -> (w108:T5)
            n163 = call-poly <vilib>:"Delacor_lib_QMH_Enqueue Message (poly).vi"("Message Data"=w108, "Message"="REQ Initialize Hardware", "Message Queue in"=w111) -> ("error out"=w104:errorcluster)  [unwired: 7 in, 1 out]
          }
          event User Event {
            # "Another Module called the \"REQ Auto setup\" API Method."
            n164 = event-data() -> ("Boolean"=w113:bool)  [unwired: 1 in]
            n165 = Bundle(cluster=T6 {"Boolean"=FALSE} ("REQ Auto setup Argument"), "Boolean"=w113) -> (w114:T6)
            n166 = call-poly <vilib>:"Delacor_lib_QMH_Enqueue Message (poly).vi"("Message Data"=w114, "Message"="REQ Auto setup", "Message Queue in"=w117) -> ("error out"=w112:errorcluster)  [unwired: 7 in, 1 out]
          }
          event User Event {
            # "Another Module called the \"Close Ref\" API Method."
            n167 = event-data() -> ("Boolean"=w119:bool)  [unwired: 1 in]
            n168 = Bundle(cluster=T7 {"Boolean"=FALSE} ("Close Ref Argument"), "Boolean"=w119) -> (w120:T7)
            n169 = call-poly <vilib>:"Delacor_lib_QMH_Enqueue Message (poly).vi"("Message Data"=w120, "Message"="Close Ref", "Message Queue in"=w123) -> ("error out"=w118:errorcluster)  [unwired: 7 in, 1 out]
          }
          event User Event {
            # "Another Module called the \"Acquire Waveform\" API Method."
            n170 = event-data() -> ("Channel"=w127:i32, "Wait Notifier"=w125:refnum<notifier>, "wait for reply"=w124:bool)  [unwired: 1 in]
            n171 = Bundle(cluster=T8 {"Channel"=0, "Wait Notifier"=refnum, "wait for reply"=FALSE} ("Acquire Waveform Argument"), "Channel"=w127, "Wait Notifier"=w125, "wait for reply"=w124) -> (w128:T8)
            n172 = call-poly <vilib>:"Delacor_lib_QMH_Enqueue Message (poly).vi"("Message Data"=w128, "Message"="Acquire Waveform", "Message Queue in"=w131) -> ("error out"=w126:errorcluster)  [unwired: 7 in, 1 out]
          }
          event User Event {
            # "Another Module called the \"REQ Channel Setting\" API Method."
            n173 = event-data() -> ("Channel Setting"=w133:T21)  [unwired: 1 in]
            n174 = Bundle(cluster=T9 {"Channel Setting"={"Channel Name (0: Channel 1)"=0, "Coupling (1: DC)"=1, "Vertical Offset (0.0)"=0.0, "Vertical Range (40.0 V)"=40.0, "Probe Attenuation (1.0)"=1.0, "Enable Channel (T: Enable)"=TRUE, "Impedance (0: 1 MOhm)"=0, "Vertical Scale (5.0 V)"=5.0, "Vertical Setting (1: Vertical Range)"=1}} ("REQ Channel Setting Argument"), "Channel Setting"=w133) -> (w134:T9)
            n175 = call-poly <vilib>:"Delacor_lib_QMH_Enqueue Message (poly).vi"("Message Data"=w134, "Message"="REQ Channel Setting", "Message Queue in"=w137) -> ("error out"=w132:errorcluster)  [unwired: 7 in, 1 out]
          }
          event User Event {
            # "Another Module called the \"REQ Configure DVM\" API Method."
            n176 = event-data() -> ("DVM Setting"=w139:T22)  [unwired: 1 in]
            n177 = Bundle(cluster=T10 {"DVM Setting"={"DVM Channel"=1, "Enable DVM Analysis"=FALSE, "Auto Range "=FALSE, "DVM Type"=0}} ("REQ Configure DVM Argument"), "DVM Setting"=w139) -> (w140:T10)
            n178 = call-poly <vilib>:"Delacor_lib_QMH_Enqueue Message (poly).vi"("Message Data"=w140, "Message"="REQ Configure DVM", "Message Queue in"=w143) -> ("error out"=w138:errorcluster)  [unwired: 7 in, 1 out]
          }
          event User Event {
            # "Another Module called the \"REQ Read DVM\" API Method."
            n179 = event-data() -> ("Wait Notifier"=w146:refnum<notifier>, "wait for reply"=w145:bool)  [unwired: 1 in]
            n180 = Bundle(cluster=T11 {"Wait Notifier"=refnum, "wait for reply"=FALSE} ("REQ Read DVM Argument"), "Wait Notifier"=w146, "wait for reply"=w145) -> (w147:T11)
            n181 = call-poly <vilib>:"Delacor_lib_QMH_Enqueue Message (poly).vi"("Message Data"=w147, "Message"="REQ Read DVM", "Message Queue in"=w150) -> ("error out"=w144:errorcluster)  [unwired: 7 in, 1 out]
          }
          event User Event {
            # "Another Module called the \"REQ Acq Waveform\" API Method."
            n182 = event-data() -> ("Boolean"=w153:bool, "Channel"=w151:i32)  [unwired: 1 in]
            n183 = Bundle(cluster=T12 {"Boolean"=FALSE, "Channel"=0} ("REQ Acq Waveform Argument"), "Boolean"=w153, "Channel"=w151) -> (w154:T12)
            n184 = call-poly <vilib>:"Delacor_lib_QMH_Enqueue Message (poly).vi"("Message Data"=w154, "Message"="REQ Acq Waveform", "Message Queue in"=w157) -> ("error out"=w152:errorcluster)  [unwired: 7 in, 1 out]
          }
          event User Event {
            # "Another Module called the \"REQ Retry Oscilloscope\" API Method."
            n185 = event-data() -> ("Boolean"=w159:bool)  [unwired: 1 in]
            n186 = Bundle(cluster=T13 {"Boolean"=FALSE} ("REQ Retry Oscilloscope Argument"), "Boolean"=w159) -> (w160:T13)
            n187 = call-poly <vilib>:"Delacor_lib_QMH_Enqueue Message (poly).vi"("Message Data"=w160, "Message"="REQ Retry Oscilloscope", "Message Queue in"=w163) -> ("error out"=w158:errorcluster)  [unwired: 7 in, 1 out]
          }
        }
        n188 = call-dynamic "Delacor_lib_QMH_Error Handler - Event Handling Loop.vi"("error in"=w54, "Message Queue in"=w48) -> ("dup error in"=w53:errorcluster)  [unwired: 8 in, 1 out]
      }
      n189 = while {
        tunnel: w33 -> [w400]
        tunnel: w35 -> [w399]
        tunnel: [w393] -> w34
        tunnel: w32 -> [w392]
        stop <- w396 stop-if-true
        n190 = Dequeue Element(queue=w399, error in (no error)=w400) -> (element=w401:T1, error out=w397:errorcluster)  [unwired: 1 in, 2 out]
        n191 = Unbundle By Name(w401) -> ("Message"=w398:string, "Data"=w395:waveform(dbl))
        n192 = case shown="\"False\", Default" w398 {
          tunnel: w397 -> [w402 w404 w406]
          tunnel: [FALSE FALSE TRUE] -> w396
          tunnel: [w402 w404 w406] -> w394
          tunnel: w395 -> [_ _ _]
          frame "False", Default {
          }
          frame "Log Data" {
          }
          frame "Stop" {
          }
        }
        n193 = call-dynamic "Delacor_lib_QMH_Error Handler - Message Handling Loop.vi"("error in"=w394, "Message Queue in"=w392) -> ("dup error in"=w393:errorcluster)  [unwired: 8 in, 1 out]
      }
    }
    frame Error {
      # "Synchronize Caller Events.vi will inform Start Module.vi that the module has launched and will let the code calling Start Module.vi register for broadcasts and would permit the caller receive the broadcast that an error occurred at launch time."
      n194 = call-dynamic "Delacor_lib_QMH_Release Message Queue.vi"("error in"=w461, "Message Queue"=w462) -> ("error out"=w460:errorcluster)  [unwired: 9 in]
      n195 = call "Synchronize Caller Events.vi"("Singleton Module Admin in"=w464) -> ("error out"=w468:errorcluster)  [unwired: 9 in, 1 out]
      n196 = call "Module Name--constant.vi"() -> ("Module Name"=w467:string)  [unwired: 11 in]
      n197 = Format Into String(format string="An error occurred during initialization. %s is no longer running.", w467) -> (resulting string=w465:string)  [unwired: 2 in, 1 out]
      n198 = Merge Errors(w460, w468) -> (w469:errorcluster)
      n199 = call "Error Reported.vi"("Additional Information"=w465, "Error"=w469) -> ()  [unwired: 9 in, 1 out]
    }
  }
  n200 = Merge Errors(w27, w30, w13) -> (w26:errorcluster)
  n201 = call "Close Module.vi"("error in (no error)"=w26, "Module Admin in"=w23) -> ("error out"=w28:errorcluster, "External Launch"=w17:bool, "Module Admin out"=w18:refnum<class "Delacor_lib_QMH_Module Admin.lvclass">)  [unwired: 7 in]
  n202 = Unregister For Events(event registration refnum=w11) -> (error out=w10:errorcluster)  [unwired: 1 in]
  n203 = Unregister For Events(event registration refnum=w22, error in=w28) -> (error out=w12:errorcluster)
  n204 = Merge Errors(w12, w10, w4) -> (→"error out":errorcluster)
  n205 = case "External Launch?" shown="True" w17 {
    tunnel: w12 -> [_ w470]
    frame False {
    }
    frame True {
      n206 = case shown="No Error" w470 {
        frame No Error {
          n207 = invoke class="VI" method="FP.Close"() -> ()  [unwired: 3 in, 3 out]
        }
        frame Error {
          n208 = invoke class="VI" method="FP.Open"("Activate"=TRUE ("Activate?")) -> ()  [unwired: 4 in, 5 out]
        }
      }
    }
  }
  n209 = local write "Module Admin"(w18) -> ()
